vi "Example 02b - Lua Scripts with Arguments.vi"() -> ()   [LabVIEW 2020]
uses:
  Lua for LabVIEW/Lua/Lua.lvclass
panel:
  out "-number":dbl
  out "-integer":i64
  out "!boolean":bool
  out "upper(string)":string
  in  "an_integer":i64=58812
  in  "a boolean":bool=TRUE
  in  "a string":string="my name is ..."
  in  "a double":dbl=2.2
  out "error out":errorcluster
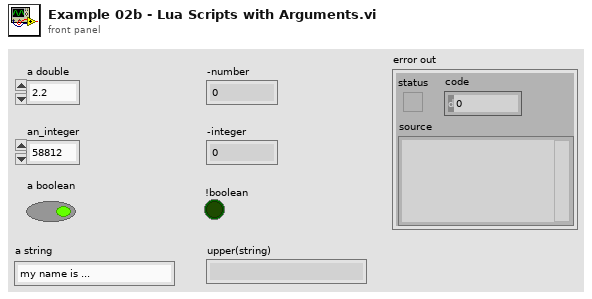
[diagram p1: front panel]
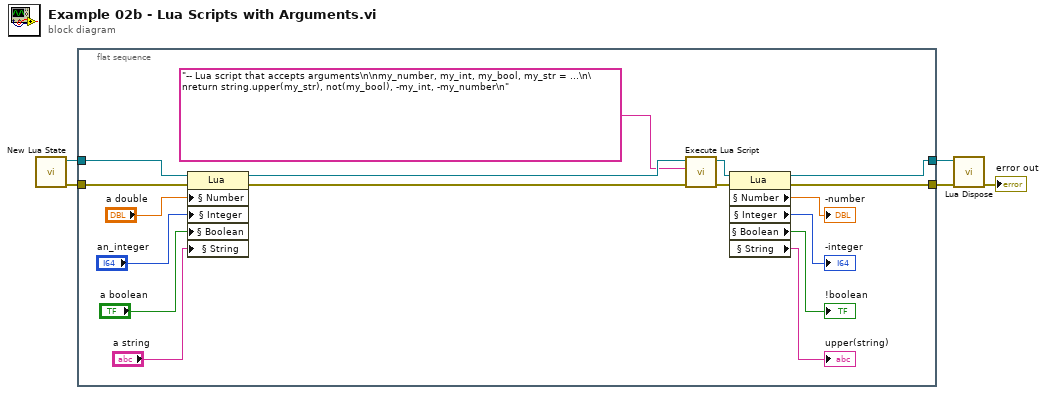
[diagram p0: block diagram]
diagram:
  n1 = call "New Lua State.vi"() -> ("error out"=w4:errorcluster, "Lua out"=w5:refnum<data-value>)  [unwired: 10 in]
  n2 = flat-sequence {
    tunnel: w5 -> [w16]
    tunnel: w4 -> [w15]
    tunnel: [w20] -> w2
    tunnel: [w19] -> w1
    frame #0 {
      n3 = property class="Lua"(reference=w16, error in=w15, "§ Number"="a double", "§ Integer"="an_integer", "§ Boolean"="a boolean", "§ String"="a string") -> (reference out=w18:refnum<data-value>, error out=w17:errorcluster)
      n4 = call "Execute Lua Script.vi"("error in (no error)"=w17, "lua script"="-- Lua script that accepts arguments\n\nmy_number, my_int, my_bool, my_str = ...\n\nreturn string.upper(my_str), not(my_bool), -my_int, -my_number\n", "Lua in"=w18) -> ("error out"=w22:errorcluster, "Lua out"=w21:refnum<data-value>)  [unwired: 7 in]
      n5 = property class="Lua"(reference=w21, error in=w22) -> (reference out=w19:refnum<data-value>, error out=w20:errorcluster, "§ Number"=→"-number":dbl, "§ Integer"=→"-integer":i64, "§ Boolean"=→"!boolean":bool, "§ String"=→"upper(string)":string)
    }
  }
  n6 = call "Lua Dispose.vi"("error in (no error)"=w2, "Disposable in"=w1) -> ("error out"=→"error out":errorcluster)  [unwired: 9 in]
